vi "Init Module.vi"(7 "Create from class input? (F)":bool, 8 "error in (no error)":errorcluster, 9 "RSI Module in":refnum<class "RSI Module.lvclass">, 10 "Slot Settings":T1, 11 "Module Model":T2) -> (0 "error out":errorcluster, 3 "RSI Module out":refnum<class "RSI Module.lvclass">)   [LabVIEW 2017, in "Modules.lvlib"]
uses:
  Modules.lvlib
  RSI Module/Module Models.ctl
  RSI Module/Slot Settings.ctl
  RSI Module/RSI Module.lvclass
  RSI Module/Channels.ctl
  RSI Module/Channel Type.ctl
  9213/9213.lvclass
  C:/Git/VeriStand/niveristand-scan-engine-module-libraries/Source/RSI Module/RSI Module.lvclass
  9203/9203.lvclass
  9205/9205.lvclass
  9207/9207.lvclass
  9211/9211.lvclass
  9212/9212.lvclass
  9214/9214.lvclass
  9217/9217.lvclass
  9219/9219.lvclass
  9229/9229.lvclass
  9233/9233.lvclass
  9234/9234.lvclass
  9235/9235.lvclass
  9237/9237.lvclass
  9239/9239.lvclass
  9242/9242.lvclass
  9244/9244.lvclass
  9401/9401.lvclass
  9402/9402.lvclass
  9403/9403.lvclass
  9478/9478.lvclass
  SD Module/SD Module.lvclass
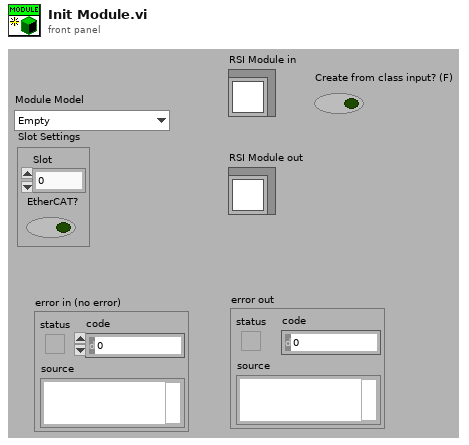
[diagram p1: front panel]
types:
  T1 = typedef "Modules.lvlib/RSI Module.lvclass/Slot Settings.ctl" = cluster{"Slot":u32, "EtherCAT?":bool}
  T2 = typedef "Modules.lvlib/RSI Module.lvclass/Module Models.ctl" = enum16{"Empty", "NI 9201", "NI 9203", "NI 9205", "NI 9206", "NI 9207", "NI 9208", "NI 9211", "NI 9212", "NI 9213", "NI 9214", "NI 9215", "NI 9217", "NI 9219", "NI 9220", "NI 9221", "NI 9222", "NI 9223", "NI 9225", "NI 9227", "NI 9229", "NI 9233", "NI 9234", "NI 9235", "NI 9236", "NI 9237", "NI 9239", "NI 9242", "NI 9244", "NI 9263", "NI 9264", "NI 9265", "NI 9266", "NI 9269", "NI 9375", "NI 9401", "NI 9402", "NI 9403", "NI 9411", "NI 9421", "NI 9422", "NI 9423", "NI 9425", "NI 9426", "NI 9435", "NI 9437", "NI 9472", "NI 9474", "NI 9475", "NI 9476", "NI 9477", "NI 9478", "NI 9481", "NI 9482", "NI 9485"}
  T3 = typedef "Modules.lvlib/RSI Module.lvclass/Channels.ctl" = cluster{"# Input Channels":i32, "# Output Channels":i32, "Channel Type":T4, "Units":string}
  T4 = typedef "Modules.lvlib/RSI Module.lvclass/Channel Type.ctl" = enum16{"Analog", "Digital"}
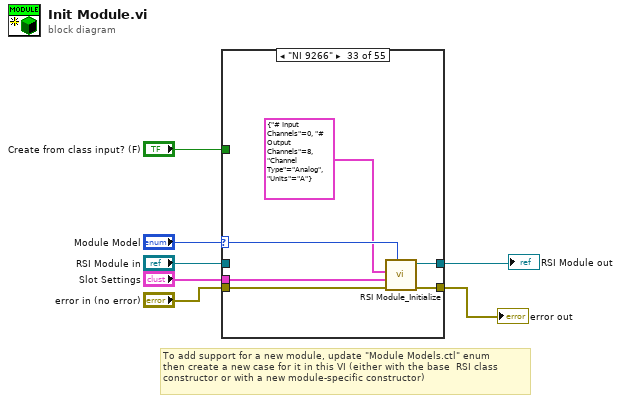
[diagram p0: block diagram]
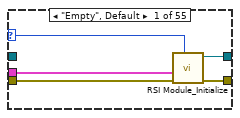
[diagram p2: hidden frame]
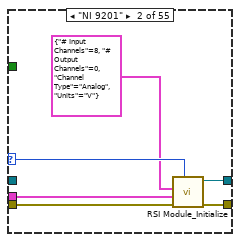
[diagram p3: hidden frame]
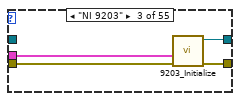
[diagram p4: hidden frame]
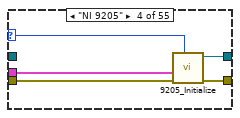
[diagram p5: hidden frame]
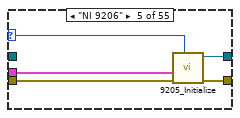
[diagram p6: hidden frame]
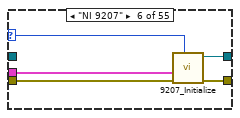
[diagram p7: hidden frame]
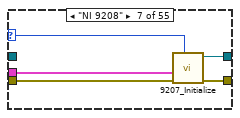
[diagram p8: hidden frame]
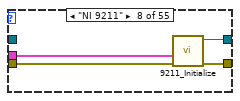
[diagram p9: hidden frame]
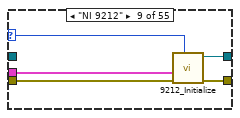
[diagram p10: hidden frame]
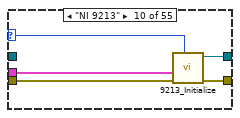
[diagram p11: hidden frame]
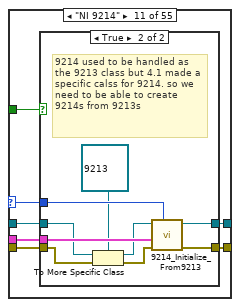
[diagram p12: hidden frame]
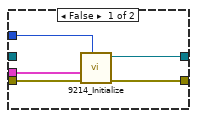
[diagram p13: hidden frame]
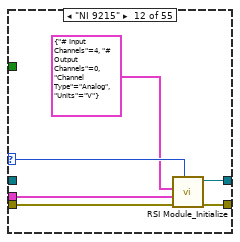
[diagram p14: hidden frame]
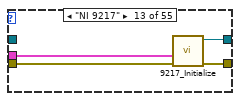
[diagram p15: hidden frame]
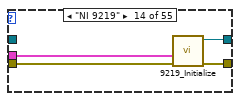
[diagram p16: hidden frame]
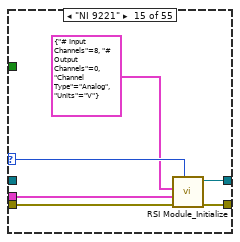
[diagram p17: hidden frame]
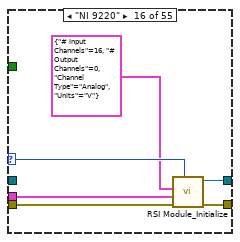
[diagram p18: hidden frame]
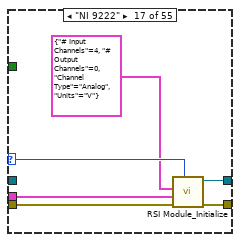
[diagram p19: hidden frame]
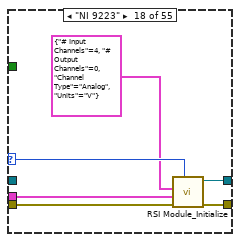
[diagram p20: hidden frame]
diagram:
  # "To add support for a new module, update \"Module Models.ctl\" enum\nthen create a new case for it in this VI (either with the base  RSI class\nconstructor or with a new module-specific constructor)"
  n1 = case shown="\"NI 9266\"" "Module Model" {
    selector: "Module Model" -> [w8 w18 _ w23 w29 w33 w38 _ w47 w52 w59 w83 _ _ w97 w103 w109 w115 w121 w127 _ _ _ w140 w145 _ _ _ _ w171 w177 w183 w189 w195 w201 _ _ _ w220 w236 w254 w274 w295 w301 w304 w324 w342 w359 w380 w402 w408 _ w418 w424 w430]
    tunnel: [w11 w17 w19 w25 w31 w35 w40 w44 w50 w55 w62 w82 w87 w91 w96 w102 w108 w114 w120 w126 w130 w134 w139 w144 w149 w151 w156 w158 w162 w170 w176 w182 w188 w194 w200 w205 w209 w213 w219 w238 w256 w276 w294 w300 w307 w326 w345 w364 w383 w401 w407 w411 w417 w423 w429] -> w3
    tunnel: [w12 w16 w22 w26 w32 w36 w41 w45 w51 w56 w63 w81 w86 w90 w95 w101 w107 w113 w119 w125 w131 w135 w138 w141 w146 w150 w157 w161 w165 w169 w175 w181 w187 w193 w199 w204 w208 w212 w218 w237 w257 w271 w293 w299 w306 w325 w344 w363 w382 w400 w406 w412 w416 w422 w428] -> w6
    tunnel: "Slot Settings" -> [w9 w14 w20 w27 w28 w37 w42 w46 w48 w53 w60 w79 w85 w89 w93 w99 w105 w111 w117 w123 w128 w133 w137 w142 w147 w152 w154 w159 w163 w167 w173 w179 w185 w191 w197 w203 w207 w211 w215 w234 w253 w273 w291 w297 w303 w322 w340 w361 w378 w398 w404 w409 w414 w420 w426]
    tunnel: "error in (no error)" -> [w10 w13 w21 w24 w30 w34 w39 w43 w49 w54 w61 w78 w84 w88 w92 w98 w104 w110 w116 w122 w129 w132 w136 w143 w148 w153 w155 w160 w164 w166 w172 w178 w184 w190 w196 w202 w206 w210 w216 w235 w252 w272 w290 w296 w302 w323 w341 w362 w379 w397 w403 w410 w413 w419 w425]
    tunnel: "Create from class input? (F)" -> [_ _ _ _ _ _ _ _ _ _ w58 _ _ _ _ _ _ _ _ _ _ _ _ _ _ _ _ _ _ _ _ _ _ _ _ _ _ _ _ _ _ _ _ _ _ _ _ _ _ _ _ _ _ _ _]
    tunnel: "RSI Module in" -> [_ _ _ _ _ _ _ _ _ _ w57 _ _ _ _ _ _ _ _ _ _ _ _ _ _ _ _ _ _ _ _ _ _ _ _ _ _ _ _ _ _ _ _ _ _ _ _ _ _ _ _ _ _ _ _]
    frame "Empty", Default {
      n2 = call "RSI Module_Initialize.vi"("Module Model"=w8, "error in (no error)"=w10, "Slot Settings"=w9) -> ("error out"=w12:errorcluster, "RSI Module out"=w11:refnum<class "RSI Module.lvclass">)  [unwired: 7 in]
    }
    frame "NI 9201" {
      n3 = call "RSI Module_Initialize.vi"("Module Model"=w18, "error in (no error)"=w13, "Slot Settings"=w14, "Channels"=T3 {"# Input Channels"=8, "# Output Channels"=0, "Channel Type"=enum."Analog", "Units"="V"}) -> ("error out"=w16:errorcluster, "RSI Module out"=w17:refnum<class "RSI Module.lvclass">)  [unwired: 6 in]
    }
    frame "NI 9203" {
      n4 = call "9203_Initialize.vi"("error in (no error)"=w21, "Slot Settings"=w20) -> ("error out"=w22:errorcluster, "9203 out"=w19:refnum<class "9203.lvclass">)  [unwired: 8 in]
    }
    frame "NI 9205" {
      n5 = call "9205_Initialize.vi"("Module Model"=w23, "error in (no error)"=w24, "Slot Settings"=w27) -> ("error out"=w26:errorcluster, "9205 out"=w25:refnum<class "9205.lvclass">)  [unwired: 7 in]
    }
    frame "NI 9206" {
      n6 = call "9205_Initialize.vi"("Module Model"=w29, "error in (no error)"=w30, "Slot Settings"=w28) -> ("error out"=w32:errorcluster, "9205 out"=w31:refnum<class "9205.lvclass">)  [unwired: 7 in]
    }
    frame "NI 9207" {
      n7 = call "9207_Initialize.vi"("Module Model"=w33, "error in (no error)"=w34, "Slot Settings"=w37) -> ("error out"=w36:errorcluster, "9207 out"=w35:refnum<class "9207.lvclass">)  [unwired: 7 in]
    }
    frame "NI 9208" {
      n8 = call "9207_Initialize.vi"("Module Model"=w38, "error in (no error)"=w39, "Slot Settings"=w42) -> ("error out"=w41:errorcluster, "9207 out"=w40:refnum<class "9207.lvclass">)  [unwired: 7 in]
    }
    frame "NI 9211" {
      n9 = call "9211_Initialize.vi"("error in (no error)"=w43, "Slot Settings"=w46) -> ("error out"=w45:errorcluster, "9211 out"=w44:refnum<class "9211.lvclass">)  [unwired: 8 in]
    }
    frame "NI 9212" {
      n10 = call "9212_Initialize.vi"("Module Model"=w47, "error in (no error)"=w49, "Slot Settings"=w48) -> ("error out"=w51:errorcluster, "9213 out"=w50:refnum<class "9212.lvclass">)  [unwired: 7 in]
    }
    frame "NI 9213" {
      n11 = call "9213_Initialize.vi"("Module Model"=w52, "error in (no error)"=w54, "Slot Settings"=w53) -> ("error out"=w56:errorcluster, "9213 out"=w55:refnum<class "9213.lvclass">)  [unwired: 7 in]
    }
    frame "NI 9214" {
      n12 = case shown="True" w58 {
        tunnel: [w68 w77] -> w63
        tunnel: [w67 w76] -> w62
        tunnel: w61 -> [w66 w73]
        tunnel: w60 -> [w65 w75]
        tunnel: w59 -> [w64 w74]
        tunnel: w57 -> [_ w72]
        frame False {
          n13 = call "9214_Initialize.vi"("Module Model"=w64, "error in (no error)"=w66, "Slot Settings"=w65) -> ("error out"=w68:errorcluster, "9214 out"=w67:refnum<class "9214.lvclass">)  [unwired: 7 in]
        }
        frame True {
          # "9214 used to be handled as the 9213 class but 4.1 made a specific calss for 9214. so we need to be able to create 9214s from 9213s"
          n14 = To More Specific Class(target class=refnum<class "9213.lvclass"> refnum ("Modules.lvlib:9213.lvclass"), reference=w72, error in=w73) -> (specific class reference=w70:refnum<class "9213.lvclass">, error out=w69:errorcluster)
          n15 = call "9214_Initialize_From9213.vi"("Module Model"=w74, "error in (no error)"=w69, "Slot Settings"=w75, "9213 in"=w70) -> ("error out"=w77:errorcluster, "9214 out"=w76:refnum<class "9214.lvclass">)  [unwired: 6 in]
        }
      }
    }
    frame "NI 9215" {
      n16 = call "RSI Module_Initialize.vi"("Module Model"=w83, "error in (no error)"=w78, "Slot Settings"=w79, "Channels"=T3 {"# Input Channels"=4, "# Output Channels"=0, "Channel Type"=enum."Analog", "Units"="V"}) -> ("error out"=w81:errorcluster, "RSI Module out"=w82:refnum<class "RSI Module.lvclass">)  [unwired: 6 in]
    }
    frame "NI 9217" {
      n17 = call "9217_Initialize.vi"("error in (no error)"=w84, "Slot Settings"=w85) -> ("error out"=w86:errorcluster, "9217 out"=w87:refnum<class "9217.lvclass">)  [unwired: 8 in]
    }
    frame "NI 9219" {
      n18 = call "9219_Initialize.vi"("error in (no error)"=w88, "Slot Settings"=w89) -> ("error out"=w90:errorcluster, "9219 out"=w91:refnum<class "9219.lvclass">)  [unwired: 8 in]
    }
    frame "NI 9221" {
      n19 = call "RSI Module_Initialize.vi"("Module Model"=w97, "error in (no error)"=w92, "Slot Settings"=w93, "Channels"=T3 {"# Input Channels"=8, "# Output Channels"=0, "Channel Type"=enum."Analog", "Units"="V"}) -> ("error out"=w95:errorcluster, "RSI Module out"=w96:refnum<class "RSI Module.lvclass">)  [unwired: 6 in]
    }
    frame "NI 9220" {
      n20 = call "RSI Module_Initialize.vi"("Module Model"=w103, "error in (no error)"=w98, "Slot Settings"=w99, "Channels"=T3 {"# Input Channels"=16, "# Output Channels"=0, "Channel Type"=enum."Analog", "Units"="V"}) -> ("error out"=w101:errorcluster, "RSI Module out"=w102:refnum<class "RSI Module.lvclass">)  [unwired: 6 in]
    }
    frame "NI 9222" {
      n21 = call "RSI Module_Initialize.vi"("Module Model"=w109, "error in (no error)"=w104, "Slot Settings"=w105, "Channels"=T3 {"# Input Channels"=4, "# Output Channels"=0, "Channel Type"=enum."Analog", "Units"="V"}) -> ("error out"=w107:errorcluster, "RSI Module out"=w108:refnum<class "RSI Module.lvclass">)  [unwired: 6 in]
    }
    frame "NI 9223" {
      n22 = call "RSI Module_Initialize.vi"("Module Model"=w115, "error in (no error)"=w110, "Slot Settings"=w111, "Channels"=T3 {"# Input Channels"=4, "# Output Channels"=0, "Channel Type"=enum."Analog", "Units"="V"}) -> ("error out"=w113:errorcluster, "RSI Module out"=w114:refnum<class "RSI Module.lvclass">)  [unwired: 6 in]
    }
    frame "NI 9225" {
      n23 = call "RSI Module_Initialize.vi"("Module Model"=w121, "error in (no error)"=w116, "Slot Settings"=w117, "Channels"=T3 {"# Input Channels"=3, "# Output Channels"=0, "Channel Type"=enum."Analog", "Units"="Vrms"}) -> ("error out"=w119:errorcluster, "RSI Module out"=w120:refnum<class "RSI Module.lvclass">)  [unwired: 6 in]
    }
    frame "NI 9227" {
      n24 = call "RSI Module_Initialize.vi"("Module Model"=w127, "error in (no error)"=w122, "Slot Settings"=w123, "Channels"=T3 {"# Input Channels"=4, "# Output Channels"=0, "Channel Type"=enum."Analog", "Units"="Arms"}) -> ("error out"=w125:errorcluster, "RSI Module out"=w126:refnum<class "RSI Module.lvclass">)  [unwired: 6 in]
    }
    frame "NI 9229" {
      n25 = call "9229_Initialize.vi"("error in (no error)"=w129, "Slot Settings"=w128) -> ("error out"=w131:errorcluster, "9229 out"=w130:refnum<class "9229.lvclass">)  [unwired: 8 in]
    }
    frame "NI 9233" {
      n26 = call "9233_Initialize.vi"("error in (no error)"=w132, "Slot Settings"=w133) -> ("error out"=w135:errorcluster, "9233 out"=w134:refnum<class "9233.lvclass">)  [unwired: 8 in]
    }
    frame "NI 9234" {
      n27 = call "9234_Initialize.vi"("error in (no error)"=w136, "Slot Settings"=w137) -> ("error out"=w138:errorcluster, "9234 out"=w139:refnum<class "9234.lvclass">)  [unwired: 8 in]
    }
    frame "NI 9235" {
      n28 = call "9235_Initialize.vi"("Module Model"=w140, "error in (no error)"=w143, "Slot Settings"=w142) -> ("error out"=w141:errorcluster, "9235 out"=w144:refnum<class "9235.lvclass">)  [unwired: 7 in]
    }
    frame "NI 9236" {
      n29 = call "9235_Initialize.vi"("Module Model"=w145, "error in (no error)"=w148, "Slot Settings"=w147) -> ("error out"=w146:errorcluster, "9235 out"=w149:refnum<class "9235.lvclass">)  [unwired: 7 in]
    }
    frame "NI 9237" {
      n30 = call "9237_Initialize.vi"("error in (no error)"=w153, "Slot Settings"=w152) -> ("error out"=w150:errorcluster, "9237 out"=w151:refnum<class "9237.lvclass">)  [unwired: 8 in]
    }
    frame "NI 9239" {
      n31 = call "9239_Initialize.vi"("error in (no error)"=w155, "Slot Settings"=w154) -> ("error out"=w157:errorcluster, "9239 out"=w156:refnum<class "9239.lvclass">)  [unwired: 8 in]
    }
    frame "NI 9242" {
      n32 = call "9242_Initialize.vi"("error in (no error)"=w160, "Slot Settings"=w159) -> ("error out"=w161:errorcluster, "Modules.lvlib:9242.lvclass"=w158:refnum<class "9242.lvclass">)  [unwired: 8 in]
    }
    frame "NI 9244" {
      n33 = call "9244_Initialize.vi"("error in (no error)"=w164, "Slot Settings"=w163) -> ("error out"=w165:errorcluster, "Modules.lvlib:9244.lvclass"=w162:refnum<class "9244.lvclass">)  [unwired: 8 in]
    }
    frame "NI 9263" {
      n34 = call "RSI Module_Initialize.vi"("Module Model"=w171, "error in (no error)"=w166, "Slot Settings"=w167, "Channels"=T3 {"# Input Channels"=0, "# Output Channels"=4, "Channel Type"=enum."Analog", "Units"="V"}) -> ("error out"=w169:errorcluster, "RSI Module out"=w170:refnum<class "RSI Module.lvclass">)  [unwired: 6 in]
    }
    frame "NI 9264" {
      n35 = call "RSI Module_Initialize.vi"("Module Model"=w177, "error in (no error)"=w172, "Slot Settings"=w173, "Channels"=T3 {"# Input Channels"=0, "# Output Channels"=16, "Channel Type"=enum."Analog", "Units"="V"}) -> ("error out"=w175:errorcluster, "RSI Module out"=w176:refnum<class "RSI Module.lvclass">)  [unwired: 6 in]
    }
    frame "NI 9265" {
      n36 = call "RSI Module_Initialize.vi"("Module Model"=w183, "error in (no error)"=w178, "Slot Settings"=w179, "Channels"=T3 {"# Input Channels"=0, "# Output Channels"=4, "Channel Type"=enum."Analog", "Units"="A"}) -> ("error out"=w181:errorcluster, "RSI Module out"=w182:refnum<class "RSI Module.lvclass">)  [unwired: 6 in]
    }
    frame "NI 9266" {
      n37 = call "RSI Module_Initialize.vi"("Module Model"=w189, "error in (no error)"=w184, "Slot Settings"=w185, "Channels"=T3 {"# Input Channels"=0, "# Output Channels"=8, "Channel Type"=enum."Analog", "Units"="A"}) -> ("error out"=w187:errorcluster, "RSI Module out"=w188:refnum<class "RSI Module.lvclass">)  [unwired: 6 in]
    }
    frame "NI 9269" {
      n38 = call "RSI Module_Initialize.vi"("Module Model"=w195, "error in (no error)"=w190, "Slot Settings"=w191, "Channels"=T3 {"# Input Channels"=0, "# Output Channels"=4, "Channel Type"=enum."Analog", "Units"="V"}) -> ("error out"=w193:errorcluster, "RSI Module out"=w194:refnum<class "RSI Module.lvclass">)  [unwired: 6 in]
    }
    frame "NI 9375" {
      n39 = call "RSI Module_Initialize.vi"("Module Model"=w201, "error in (no error)"=w196, "Slot Settings"=w197, "Channels"=T3 {"# Input Channels"=16, "# Output Channels"=16, "Channel Type"=enum."Digital", "Units"=""}) -> ("error out"=w199:errorcluster, "RSI Module out"=w200:refnum<class "RSI Module.lvclass">)  [unwired: 6 in]
    }
    frame "NI 9401" {
      n40 = call "9401_Initialize.vi"("error in (no error)"=w202, "Slot Settings"=w203) -> ("error out"=w204:errorcluster, "9401 out"=w205:refnum<class "9401.lvclass">)  [unwired: 8 in]
    }
    frame "NI 9402" {
      n41 = call "9402_Initialize.vi"("error in (no error)"=w206, "Slot Settings"=w207) -> ("error out"=w208:errorcluster, "9402 out"=w209:refnum<class "9402.lvclass">)  [unwired: 8 in]
    }
    frame "NI 9403" {
      n42 = call "9403_Initialize.vi"("error in (no error)"=w210, "Slot Settings"=w211) -> ("error out"=w212:errorcluster, "9403 out"=w213:refnum<class "9403.lvclass">)  [unwired: 8 in]
    }
    frame "NI 9411" {
      n43 = Unbundle By Name(w215) -> ("EtherCAT?"=w214:bool)
      n44 = case shown="True" w214 {
        tunnel: w220 -> [w226 w229]
        tunnel: [w225 w230] -> w219
        tunnel: [w224 w231] -> w218
        tunnel: T3 {"# Input Channels"=6, "# Output Channels"=0, "Channel Type"=enum."Digital", "Units"=""} ("Channels") -> [w223 w228]
        tunnel: w216 -> [w222 w232]
        tunnel: w215 -> [w221 w227]
        frame False {
          n45 = call "SD Module_Initialize.vi"("Module Model"=w226, "error in (no error)"=w222, "Slot Settings"=w221, "Channels"=w223) -> ("error out"=w224:errorcluster, "SD Module out"=w225:refnum<class "SD Module.lvclass">)  [unwired: 6 in]
        }
        frame True {
          n46 = call "RSI Module_Initialize.vi"("Module Model"=w229, "error in (no error)"=w232, "Slot Settings"=w227, "Channels"=w228) -> ("error out"=w231:errorcluster, "RSI Module out"=w230:refnum<class "RSI Module.lvclass">)  [unwired: 6 in]
        }
      }
    }
    frame "NI 9421" {
      n47 = Unbundle By Name(w234) -> ("EtherCAT?"=w239:bool)
      n48 = case shown="True" w239 {
        tunnel: w236 -> [w245 w248]
        tunnel: [w244 w249] -> w238
        tunnel: [w243 w250] -> w237
        tunnel: T3 {"# Input Channels"=8, "# Output Channels"=0, "Channel Type"=enum."Digital", "Units"=""} ("Channels") -> [w242 w247]
        tunnel: w235 -> [w241 w251]
        tunnel: w234 -> [w240 w246]
        frame False {
          n49 = call "SD Module_Initialize.vi"("Module Model"=w245, "error in (no error)"=w241, "Slot Settings"=w240, "Channels"=w242) -> ("error out"=w243:errorcluster, "SD Module out"=w244:refnum<class "SD Module.lvclass">)  [unwired: 6 in]
        }
        frame True {
          n50 = call "RSI Module_Initialize.vi"("Module Model"=w248, "error in (no error)"=w251, "Slot Settings"=w246, "Channels"=w247) -> ("error out"=w250:errorcluster, "RSI Module out"=w249:refnum<class "RSI Module.lvclass">)  [unwired: 6 in]
        }
      }
    }
    frame "NI 9422" {
      n51 = Unbundle By Name(w253) -> ("EtherCAT?"=w258:bool)
      n52 = case shown="True" w258 {
        tunnel: w254 -> [w264 w267]
        tunnel: [w263 w268] -> w256
        tunnel: [w262 w269] -> w257
        tunnel: T3 {"# Input Channels"=8, "# Output Channels"=0, "Channel Type"=enum."Digital", "Units"=""} ("Channels") -> [w261 w266]
        tunnel: w252 -> [w260 w270]
        tunnel: w253 -> [w259 w265]
        frame False {
          n53 = call "SD Module_Initialize.vi"("Module Model"=w264, "error in (no error)"=w260, "Slot Settings"=w259, "Channels"=w261) -> ("error out"=w262:errorcluster, "SD Module out"=w263:refnum<class "SD Module.lvclass">)  [unwired: 6 in]
        }
        frame True {
          n54 = call "RSI Module_Initialize.vi"("Module Model"=w267, "error in (no error)"=w270, "Slot Settings"=w265, "Channels"=w266) -> ("error out"=w269:errorcluster, "RSI Module out"=w268:refnum<class "RSI Module.lvclass">)  [unwired: 6 in]
        }
      }
    }
    frame "NI 9423" {
      n55 = Unbundle By Name(w273) -> ("EtherCAT?"=w277:bool)
      n56 = case shown="False" w277 {
        tunnel: w274 -> [w283 w286]
        tunnel: [w282 w287] -> w276
        tunnel: [w281 w288] -> w271
        tunnel: T3 {"# Input Channels"=8, "# Output Channels"=0, "Channel Type"=enum."Digital", "Units"=""} ("Channels") -> [w280 w285]
        tunnel: w272 -> [w279 w289]
        tunnel: w273 -> [w278 w284]
        frame False {
          n57 = call "SD Module_Initialize.vi"("Module Model"=w283, "error in (no error)"=w279, "Slot Settings"=w278, "Channels"=w280) -> ("error out"=w281:errorcluster, "SD Module out"=w282:refnum<class "SD Module.lvclass">)  [unwired: 6 in]
        }
        frame True {
          n58 = call "RSI Module_Initialize.vi"("Module Model"=w286, "error in (no error)"=w289, "Slot Settings"=w284, "Channels"=w285) -> ("error out"=w288:errorcluster, "RSI Module out"=w287:refnum<class "RSI Module.lvclass">)  [unwired: 6 in]
        }
      }
    }
    frame "NI 9425" {
      n59 = call "RSI Module_Initialize.vi"("Module Model"=w295, "error in (no error)"=w290, "Slot Settings"=w291, "Channels"=T3 {"# Input Channels"=32, "# Output Channels"=0, "Channel Type"=enum."Digital", "Units"=""}) -> ("error out"=w293:errorcluster, "RSI Module out"=w294:refnum<class "RSI Module.lvclass">)  [unwired: 6 in]
    }
    frame "NI 9426" {
      n60 = call "RSI Module_Initialize.vi"("Module Model"=w301, "error in (no error)"=w296, "Slot Settings"=w297, "Channels"=T3 {"# Input Channels"=32, "# Output Channels"=0, "Channel Type"=enum."Digital", "Units"=""}) -> ("error out"=w299:errorcluster, "RSI Module out"=w300:refnum<class "RSI Module.lvclass">)  [unwired: 6 in]
    }
    frame "NI 9435" {
      n61 = Unbundle By Name(w303) -> ("EtherCAT?"=w308:bool)
      n62 = case shown="True" w308 {
        tunnel: w304 -> [w314 w317]
        tunnel: [w313 w318] -> w307
        tunnel: [w312 w319] -> w306
        tunnel: T3 {"# Input Channels"=4, "# Output Channels"=0, "Channel Type"=enum."Digital", "Units"=""} ("Channels") -> [w311 w316]
        tunnel: w302 -> [w310 w320]
        tunnel: w303 -> [w309 w315]
        frame False {
          n63 = call "SD Module_Initialize.vi"("Module Model"=w314, "error in (no error)"=w310, "Slot Settings"=w309, "Channels"=w311) -> ("error out"=w312:errorcluster, "SD Module out"=w313:refnum<class "SD Module.lvclass">)  [unwired: 6 in]
        }
        frame True {
          n64 = call "RSI Module_Initialize.vi"("Module Model"=w317, "error in (no error)"=w320, "Slot Settings"=w315, "Channels"=w316) -> ("error out"=w319:errorcluster, "RSI Module out"=w318:refnum<class "RSI Module.lvclass">)  [unwired: 6 in]
        }
      }
    }
    frame "NI 9437" {
      n65 = Unbundle By Name(w322) -> ("EtherCAT?"=w327:bool)
      n66 = case shown="False" w327 {
        tunnel: w324 -> [w333 w336]
        tunnel: [w332 w337] -> w326
        tunnel: [w331 w338] -> w325
        tunnel: T3 {"# Input Channels"=8, "# Output Channels"=0, "Channel Type"=enum."Digital", "Units"=""} ("Channels") -> [w330 w335]
        tunnel: w323 -> [w329 w339]
        tunnel: w322 -> [w328 w334]
        frame False {
          n67 = call "SD Module_Initialize.vi"("Module Model"=w333, "error in (no error)"=w329, "Slot Settings"=w328, "Channels"=w330) -> ("error out"=w331:errorcluster, "SD Module out"=w332:refnum<class "SD Module.lvclass">)  [unwired: 6 in]
        }
        frame True {
          n68 = call "RSI Module_Initialize.vi"("Module Model"=w336, "error in (no error)"=w339, "Slot Settings"=w334, "Channels"=w335) -> ("error out"=w338:errorcluster, "RSI Module out"=w337:refnum<class "RSI Module.lvclass">)  [unwired: 6 in]
        }
      }
    }
    frame "NI 9472" {
      n69 = Unbundle By Name(w340) -> ("EtherCAT?"=w346:bool)
      n70 = case shown="True" w346 {
        tunnel: w342 -> [w352 w355]
        tunnel: [w351 w356] -> w345
        tunnel: [w350 w357] -> w344
        tunnel: T3 {"# Input Channels"=0, "# Output Channels"=8, "Channel Type"=enum."Digital", "Units"=""} ("Channels") -> [w349 w354]
        tunnel: w341 -> [w348 w358]
        tunnel: w340 -> [w347 w353]
        frame False {
          n71 = call "SD Module_Initialize.vi"("Module Model"=w352, "error in (no error)"=w348, "Slot Settings"=w347, "Channels"=w349) -> ("error out"=w350:errorcluster, "SD Module out"=w351:refnum<class "SD Module.lvclass">)  [unwired: 6 in]
        }
        frame True {
          n72 = call "RSI Module_Initialize.vi"("Module Model"=w355, "error in (no error)"=w358, "Slot Settings"=w353, "Channels"=w354) -> ("error out"=w357:errorcluster, "RSI Module out"=w356:refnum<class "RSI Module.lvclass">)  [unwired: 6 in]
        }
      }
    }
    frame "NI 9474" {
      n73 = Unbundle By Name(w361) -> ("EtherCAT?"=w365:bool)
      n74 = case shown="False" w365 {
        tunnel: w359 -> [w371 w374]
        tunnel: [w370 w375] -> w364
        tunnel: [w369 w376] -> w363
        tunnel: T3 {"# Input Channels"=0, "# Output Channels"=8, "Channel Type"=enum."Digital", "Units"=""} ("Channels") -> [w368 w373]
        tunnel: w362 -> [w367 w377]
        tunnel: w361 -> [w366 w372]
        frame False {
          n75 = call "SD Module_Initialize.vi"("Module Model"=w371, "error in (no error)"=w367, "Slot Settings"=w366, "Channels"=w368) -> ("error out"=w369:errorcluster, "SD Module out"=w370:refnum<class "SD Module.lvclass">)  [unwired: 6 in]
        }
        frame True {
          n76 = call "RSI Module_Initialize.vi"("Module Model"=w374, "error in (no error)"=w377, "Slot Settings"=w372, "Channels"=w373) -> ("error out"=w376:errorcluster, "RSI Module out"=w375:refnum<class "RSI Module.lvclass">)  [unwired: 6 in]
        }
      }
    }
    frame "NI 9475" {
      n77 = Unbundle By Name(w378) -> ("EtherCAT?"=w384:bool)
      n78 = case shown="True" w384 {
        tunnel: w380 -> [w390 w393]
        tunnel: [w389 w394] -> w383
        tunnel: [w388 w395] -> w382
        tunnel: T3 {"# Input Channels"=0, "# Output Channels"=8, "Channel Type"=enum."Digital", "Units"=""} ("Channels") -> [w387 w392]
        tunnel: w379 -> [w386 w396]
        tunnel: w378 -> [w385 w391]
        frame False {
          n79 = call "SD Module_Initialize.vi"("Module Model"=w390, "error in (no error)"=w386, "Slot Settings"=w385, "Channels"=w387) -> ("error out"=w388:errorcluster, "SD Module out"=w389:refnum<class "SD Module.lvclass">)  [unwired: 6 in]
        }
        frame True {
          n80 = call "RSI Module_Initialize.vi"("Module Model"=w393, "error in (no error)"=w396, "Slot Settings"=w391, "Channels"=w392) -> ("error out"=w395:errorcluster, "RSI Module out"=w394:refnum<class "RSI Module.lvclass">)  [unwired: 6 in]
        }
      }
    }
    frame "NI 9476" {
      n81 = call "RSI Module_Initialize.vi"("Module Model"=w402, "error in (no error)"=w397, "Slot Settings"=w398, "Channels"=T3 {"# Input Channels"=0, "# Output Channels"=32, "Channel Type"=enum."Digital", "Units"=""}) -> ("error out"=w400:errorcluster, "RSI Module out"=w401:refnum<class "RSI Module.lvclass">)  [unwired: 6 in]
    }
    frame "NI 9477" {
      n82 = call "RSI Module_Initialize.vi"("Module Model"=w408, "error in (no error)"=w403, "Slot Settings"=w404, "Channels"=T3 {"# Input Channels"=0, "# Output Channels"=32, "Channel Type"=enum."Digital", "Units"=""}) -> ("error out"=w406:errorcluster, "RSI Module out"=w407:refnum<class "RSI Module.lvclass">)  [unwired: 6 in]
    }
    frame "NI 9478" {
      n83 = call "9478_Initialize.vi"("error in (no error)"=w410, "Slot Settings"=w409) -> ("error out"=w412:errorcluster, "9478 out"=w411:refnum<class "9478.lvclass">)  [unwired: 8 in]
    }
    frame "NI 9481" {
      n84 = call "RSI Module_Initialize.vi"("Module Model"=w418, "error in (no error)"=w413, "Slot Settings"=w414, "Channels"=T3 {"# Input Channels"=0, "# Output Channels"=4, "Channel Type"=enum."Digital", "Units"=""}) -> ("error out"=w416:errorcluster, "RSI Module out"=w417:refnum<class "RSI Module.lvclass">)  [unwired: 6 in]
    }
    frame "NI 9482" {
      n85 = call "RSI Module_Initialize.vi"("Module Model"=w424, "error in (no error)"=w419, "Slot Settings"=w420, "Channels"=T3 {"# Input Channels"=0, "# Output Channels"=4, "Channel Type"=enum."Digital", "Units"=""}) -> ("error out"=w422:errorcluster, "RSI Module out"=w423:refnum<class "RSI Module.lvclass">)  [unwired: 6 in]
    }
    frame "NI 9485" {
      n86 = call "RSI Module_Initialize.vi"("Module Model"=w430, "error in (no error)"=w425, "Slot Settings"=w426, "Channels"=T3 {"# Input Channels"=0, "# Output Channels"=8, "Channel Type"=enum."Digital", "Units"=""}) -> ("error out"=w428:errorcluster, "RSI Module out"=w429:refnum<class "RSI Module.lvclass">)  [unwired: 6 in]
    }
  }
  "error out" <- w6
  "RSI Module out" <- w3
